vi "ex2_3.vi"() -> ()   [LabVIEW 2017]
panel:
  in  "Known resistance":dbl
  out "Unknown resistance":dbl
  in  "stop":bool
  out "Measured voltage":dbl
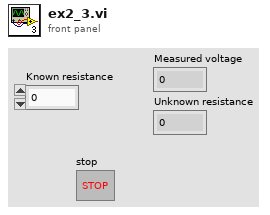
[diagram p1: front panel]
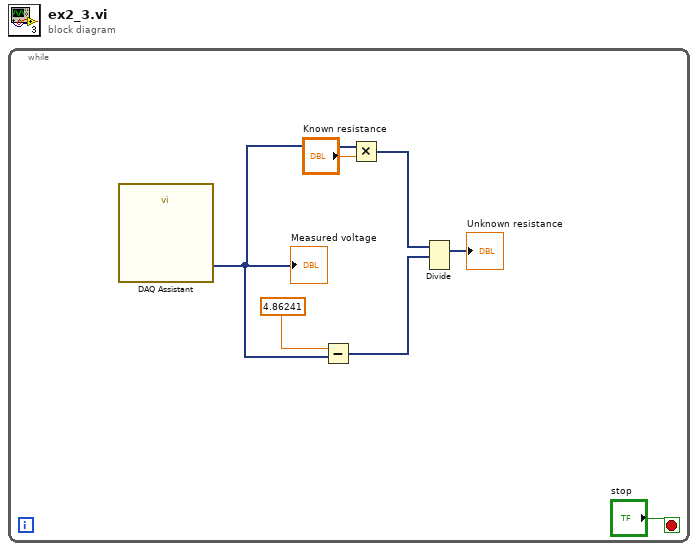
[diagram p0: block diagram]
diagram:
  n1 = while {
    stop <- "stop" stop-if-true
    n2 = call "DAQ Assistant"() -> ("data"=w5:dynamicdata)  [unwired: 17 in, 2 out]
    "Measured voltage" <- w5
    n3 = Subtract(x=4.86241, y=w5) -> (x-y=w3:dynamicdata)
    n4 = Multiply(x=w5, y="Known resistance") -> (x*y=w4:dynamicdata)
    n5 = Divide(1:w3, 2:w4) -> (0:→"Unknown resistance":dynamicdata)  [unwired: 1 in, 1 out]
  }
